vi "Update Case Frame to Image.vi"(4 "Zoom Factor":sgl=1.0, 5 "Picture Control Reference":refnum<vi>, 6 "Config Path (\"\" For Lvcsm File)":path, 7 "Application Reference (Local)":refnum<vi>, 8 "error in (no error)":errorcluster, 9 "Type":enum16{"CSM", "CSM-VI"}(ring), 10 "State":string, 11 "Name":string) -> (0 "Error Out":errorcluster, 2 "New Picture":picture)   [LabVIEW 2017, in "CSM-Helper API with lvcsm Support.lvlib"]
uses:
  CSM-Helper API with lvcsm Support.lvlib
  CSM-Helper.lvclass/CSM-Helper.ctl
  4183b97d-67e9-48d0-9013-287ea012034b.vi
  901ca4ca-129f-45f5-aaf1-2c7f5df1094f.vi
  Properties/Read Case Structure Ref.vi
  API/Destroy.vi
  API/Get CaseFrame Index By CaseName.vi
  API/Create From VI Reference.vi
  lvcsmFile/_Array of VData to VCluster.vi
  <vilib>/Utility/config.llb/Close Config Data.vi
  <vilib>/Utility/config.llb/Read Key.vi
  <vilib>/Utility/config.llb/Read Key (Double).vi
  <vilib>/Utility/config.llb/Read Key (I32).vi
  lvcsmFile/lvcsm String to Path.vi
  <vilib>/Utility/config.llb/Read Key (String).vi
  lvcsmFile/Path to lvcsm String.vi
  <vilib>/Utility/config.llb/Get Key Names.vi
  <vilib>/Utility/Data Type/Get Type Information.vi
  <vilib>/Utility/Data Type/Get Array Information.vi
  <vilib>/Utility/config.llb/Read Key (Boolean).vi
  <vilib>/Utility/config.llb/Open Config Data.vi
  lvcsmFile/lvcsm File Path.vi
  CSM-Helper.lvclass
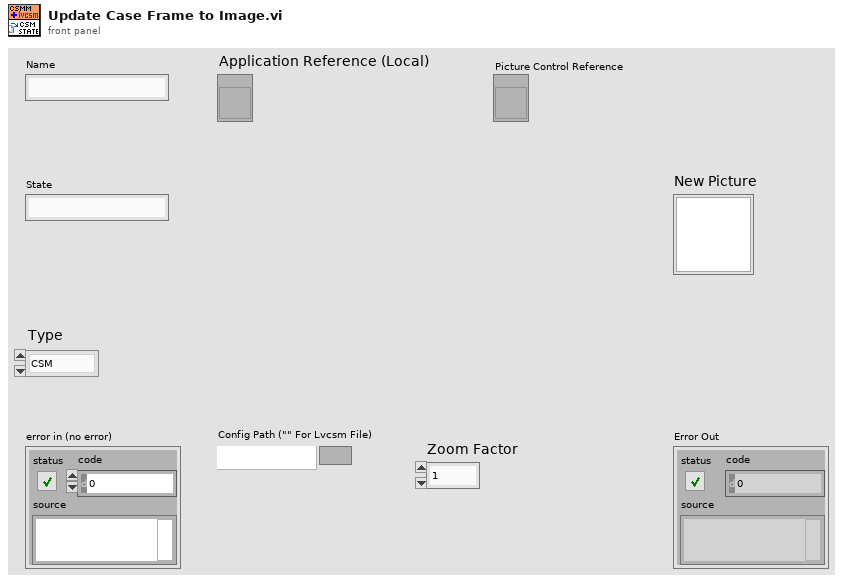
[diagram p1: front panel]
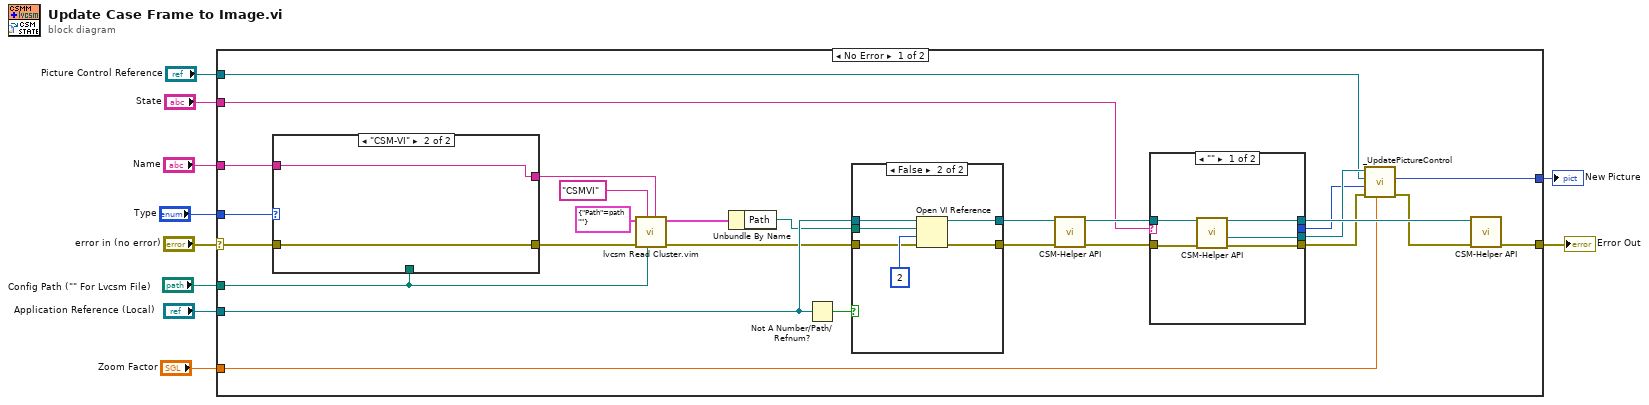
[diagram p0: block diagram]
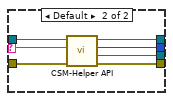
[diagram p2: hidden frame]
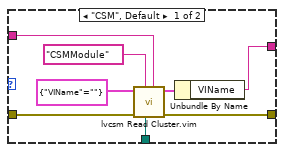
[diagram p3: hidden frame]
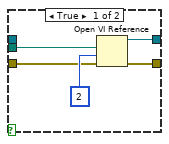
[diagram p4: hidden frame]
diagram:
  n1 = case shown="No Error" "error in (no error)" {
    selector: "error in (no error)" -> [w37 w71]
    tunnel: [w29 w71] -> w10
    tunnel: "Name" -> [w36 _]
    tunnel: "Config Path (\"\" For Lvcsm File)" -> [w20 _]
    tunnel: "State" -> [w31 _]
    tunnel: "Application Reference (Local)" -> [w28 _]
    tunnel: "Type" -> [w18 _]
    tunnel: "Picture Control Reference" -> [w13 _]
    tunnel: [w12 _] -> w2
    tunnel: "Zoom Factor" -> [w11 _]
    frame No Error {
      n2 = case shown="\"CSM-VI\"" w18 {
        tunnel: w37 -> [w57 w59]
        tunnel: w36 -> [w55 w58]
        tunnel: [w52 w58] -> w23
        tunnel: [w51 w59] -> w21
        tunnel: w20 -> [w50 _]
        frame "CSM", Default {
          n3 = call "lvcsm Read Cluster.vim"("Sub-section (\"\")"=w55, "Config Path"=w50, "Section"="CSMModule", "Error In"=w57, "Default Prototype"=cluster{"VIName":string} {"VIName"=""}) -> ("error out"=w51:errorcluster, "Cluster (Dup)"=w53:cluster{"VIName":string})  [unwired: 5 in]
          n4 = Unbundle By Name(w53) -> ("VIName"=w52:string)
        }
        frame "CSM-VI" {
        }
      }
      n5 = call "lvcsm Read Cluster.vim"("Sub-section (\"\")"=w23, "Config Path"=w20, "Section"="CSMVI", "Error In"=w21, "Default Prototype"=cluster{"Path":path} {"Path"=path ""}) -> ("error out"=w22:errorcluster, "Cluster (Dup)"=w26:cluster{"Path":path})  [unwired: 5 in]
      n6 = Unbundle By Name(w26) -> ("Path"=w19:path)
      n7 = Not A Number/Path/Refnum?(number/path/refnum=w28) -> (NaN/Path/Refnum?=w27:bool)
      n8 = case shown="False" w27 {
        tunnel: [w64 w70] -> w35
        tunnel: [w63 w69] -> w34
        tunnel: w22 -> [w61 w67]
        tunnel: w28 -> [_ w66]
        tunnel: w19 -> [w60 w65]
        frame True {
          n9 = Open VI Reference(vi path=w60, options=2, error in (no error)=w61) -> (vi reference=w63:refnum<vi>, error out=w64:errorcluster)  [unwired: 3 in]
        }
        frame False {
          n10 = Open VI Reference(application reference (local)=w66, vi path=w65, options=2, error in (no error)=w67) -> (vi reference=w69:refnum<vi>, error out=w70:errorcluster)  [unwired: 2 in]
        }
      }
      n11 = call-poly "CSM-Helper API.vi"("error in (no error)"=w35, "VI"=w34) -> ("error out"=w33:errorcluster, "CSM-Helper.lvclass"=w32:refnum<class "CSM-Helper.lvclass">)  [unwired: 8 in]
      n12 = case shown="\"\"" w31 {
        selector: w31 -> [_ w47]
        tunnel: w33 -> [w42 w49]
        tunnel: w32 -> [w41 w48]
        tunnel: [w38 w46] -> w30
        tunnel: [w39 w45] -> w17
        tunnel: [w40 w44] -> w15
        tunnel: [_ w43] -> w14
        frame "" {
          n13 = call-poly "CSM-Helper API.vi"("error in (no error)"=w42, "CSM-Helper in"=w41) -> ("error out"=w39:errorcluster, "Case Structure"=w40:refnum<vi>, "CSM-Helper out"=w38:refnum<class "CSM-Helper.lvclass">)  [unwired: 7 in]
        }
        frame Default {
          n14 = call-poly "CSM-Helper API.vi"("error in (no error)"=w49, "CASE"=w47, "CSM-Helper in"=w48) -> ("error out"=w45:errorcluster, "CaseStruRef"=w44:refnum<vi>, "index"=w43:i32, "CSM-Helper out"=w46:refnum<class "CSM-Helper.lvclass">)  [unwired: 5 in]
        }
      }
      n15 = call "_UpdatePictureControl.vi"("Zoom Factor"=w11, "error in (no error)"=w17, "Visible Frame"=w14, "Picture Control Reference"=w13, "Center Object Reference"=w15) -> ("error out"=w16:errorcluster, "New Picture"=w12:picture)  [unwired: 5 in]
      n16 = call-poly "CSM-Helper API.vi"("error in (no error)"=w16, "CSM-Helper in"=w30) -> ("error out"=w29:errorcluster)  [unwired: 8 in, 1 out]
    }
    frame Error {
    }
  }
  "Error Out" <- w10
  "New Picture" <- w2
